vi "CheckDiskSpace.vi"(8 "error in (no error)":errorcluster, 11 "minimum free disk space":i32) -> (0 "error out":errorcluster, 1 "available disk space":bool, 2 "free disk space":dbl, 3 "data directory":path)   [LabVIEW 2017, in "FileManager.lvlib"]
uses:
  <vilib>/addons/InsightCM/Devices/Shared/Common/FileManager/FileManager.lvlib
  <vilib>/addons/InsightCM/Utilities/GlobalConfiguration/GlobalConfiguration.lvlib
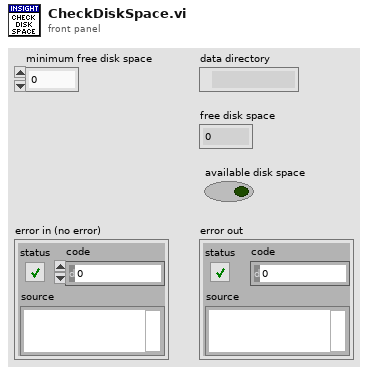
[diagram p1: front panel]
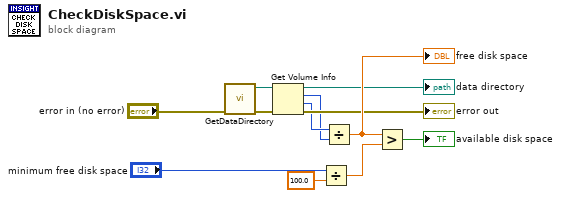
[diagram p0: block diagram]
diagram:
  n1 = call <vilib>:"GetDataDirectory.vi"("error in (no error)"="error in (no error)") -> ("error out"=w2:errorcluster, "data directory"=w3:path)  [unwired: 9 in]
  n2 = Get Volume Info(8:w2, 11:w3) -> (0:→"error out":errorcluster, 1:w4:i64, 2:w1:i64, 3:→"data directory":path)  [unwired: 2 out]
  n3 = Divide(x="minimum free disk space", y=100.0) -> (x/y=w9:dbl)
  n4 = Divide(x=w4, y=w1) -> (x/y=w12:dbl)
  "free disk space" <- w12
  n5 = Greater?(x=w12, y=w9) -> (0:→"available disk space":bool)
